vi "TestData_Text2SQL.vi"(8 "error in (no error)":errorcluster caption="错误输入（无错误）", 10 "Record_Text":string, 11 "SQL File":path) -> (0 "error out":errorcluster caption="错误输出", 1 "Hash_Code":string, 2 "SQL Outpout":string, 3 "ok?":bool)   [LabVIEW 2012, in "Lib_UEL.ATE.lvlib" / "Lib_TestData.lvlib"]
uses:
  Lib_TestData.lvlib
  <vilib>/Utility/config.llb/Read Key (String).vi
  <vilib>/Utility/config.llb/NI_LVConfig.lvlib
panel:
  # "功能说明:\n- 将一条记录的表格字符串转换为可以直接执行的 SQL INSERT语句.\n- 兼容不同的分隔符.\n- 兼容已知的错误格式\n---- spare1~4列,没有 \n\n插入语句标准: 留意转换后最后一列为空.\n- 255列, 以#分隔, \n- 251列, 以#分隔, 缺少: No47记录后,spare1~4列\n- 添加最后一列: hash列"
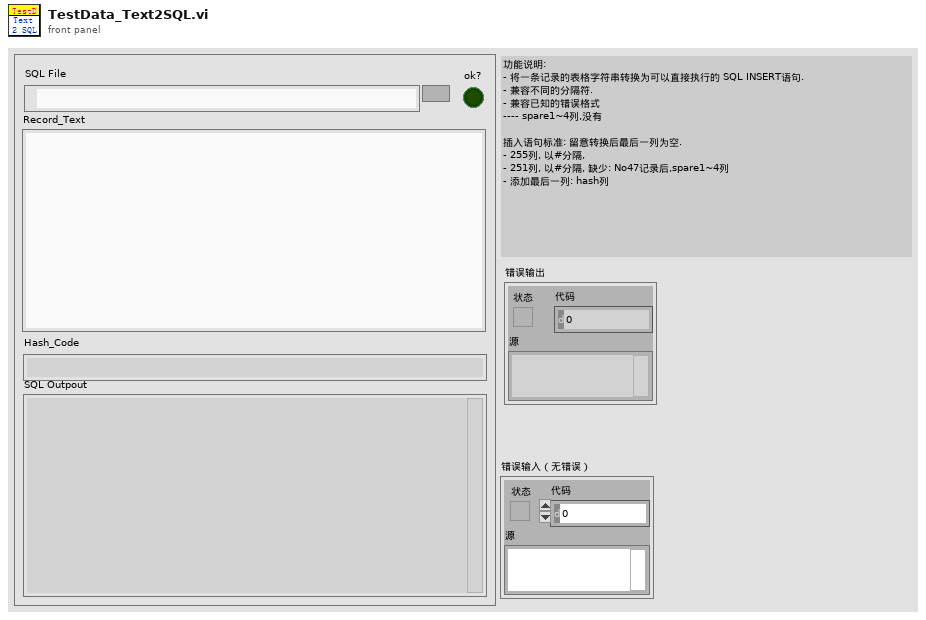
[diagram p1: front panel]
types:
  T1 = typedef "NI_LVConfig.lvlib/Config Data RefNum.ctl" = refnum<k1>
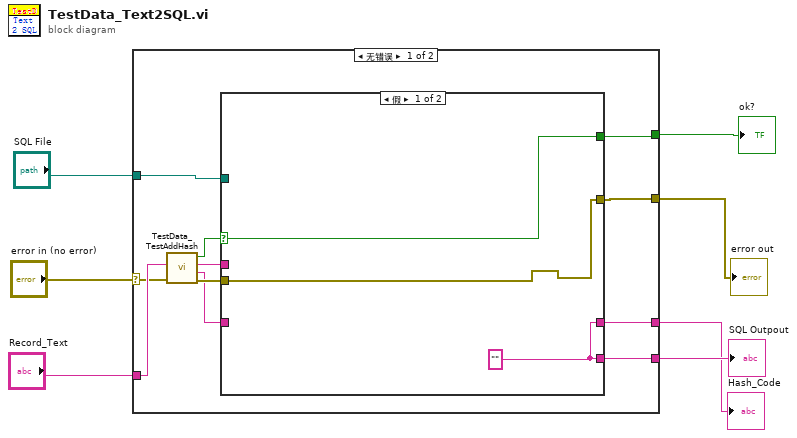
[diagram p0: block diagram]
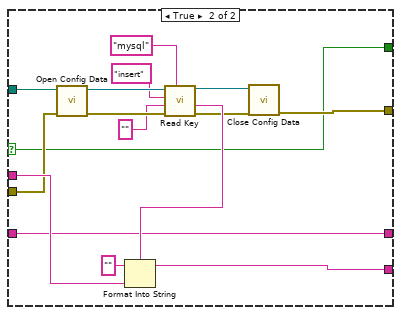
[diagram p2: hidden frame]
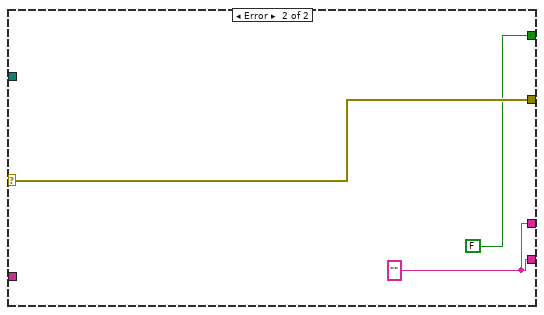
[diagram p3: hidden frame]
diagram:
  n1 = case shown="无错误" "error in (no error)" {
    selector: "error in (no error)" -> [w15 w40]
    tunnel: "SQL File" -> [w18 _]
    tunnel: [w12 w40] -> w5
    tunnel: [w10 FALSE ("ok?")] -> w4
    tunnel: "Record_Text" -> [w16 _]
    tunnel: [w17 w38] -> w2
    tunnel: [w9 w38] -> w1
    frame No Error {
      n2 = call "TestData_TestAddHash.vi"("error in (no error)"=w15, "Record_Text"=w16) -> ("error out"=w13:errorcluster, "Hash_Code"=w8:string, "RecordText Outpout"=w14:string, "ok?"=w11:bool)  [unwired: 6 in]
      n3 = case shown="假" w11 {
        selector: w11 -> [w21 w23]
        tunnel: w18 -> [_ w37]
        tunnel: [w19 w36] -> w17
        tunnel: w14 -> [_ w33]
        tunnel: w13 -> [w20 w32]
        tunnel: [w20 w31] -> w12
        tunnel: [w21 w23] -> w10
        tunnel: [w19 w22] -> w9
        tunnel: w8 -> [_ w22]
        frame False {
          w19 = ""
        }
        frame True {
          n4 = call <vilib>:"Open Config Data.vi"("error in (no error)"=w32, "configuration file path"=w37) -> ("error out"=w30:errorcluster, "refnum"=w29:T1)  [unwired: 7 in, 1 out]
          n5 = call-poly <vilib>:"Read Key.vi"("section"="mysql", "error in (no error)"=w30, "default value"="", "key"="insert", "refnum"=w29) -> ("error out"=w25:errorcluster, "value"=w35:string, "refnum out"=w24:T1)  [unwired: 3 in, 1 out]
          n6 = Format Into String(format string=w35, initial string="" ("初始字符串"), w33) -> (resulting string=w36:string)  [unwired: 1 in, 1 out]
          n7 = call <vilib>:"Close Config Data.vi"("error in (no error)"=w25, "refnum"=w24) -> ("error out"=w31:errorcluster)  [unwired: 8 in, 1 out]
        }
      }
    }
    frame Error {
      w38 = "" ("SQL Outpout")
    }
  }
  "ok?" <- w4
  "SQL Outpout" <- w2
  "error out" <- w5
  "Hash_Code" <- w1
